vi "toMsgQueue.vi"(8 "error in":errorcluster, 11 "ITaskChannel":refnum<class "ITaskChannel.lvclass">) -> (0 "error out":errorcluster, 3 "queueRef":refnum<queue>)   [LabVIEW 2023, in "TLC_Daemon.lvlib"]
uses:
  TLC_Daemon.lvlib
  ITaskChannel/ITaskChannel.lvclass
  Ctrls/msg.ctl
  MsgQueueTaskChannel/MsgQueueTaskChannel.lvclass
  MsgQueueTaskChannel/Read queueRef.vi
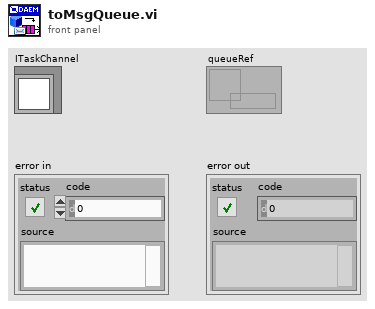
[diagram p1: front panel]
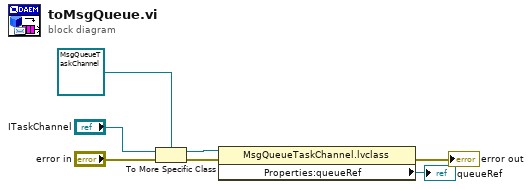
[diagram p0: block diagram]
diagram:
  n1 = To More Specific Class(target class=refnum<class "MsgQueueTaskChannel.lvclass"> refnum ("TLC_Daemon.lvlib:MsgQueueTaskChannel.lvclass"), reference="ITaskChannel", error in="error in") -> (specific class reference=w5:refnum<class "MsgQueueTaskChannel.lvclass">, error out=w6:errorcluster)
  n2 = property class="MsgQueueTaskChannel.lvclass"(reference=w5, error in=w6) -> (error out=→"error out":errorcluster, "Properties:queueRef"=→"queueRef":refnum<queue>)  [unwired: 1 out]
